vi "JogParams_KCubeInertial.vi"(6 "JogMode in":i32, 9 "JogAcceleration in":i32, 10 "JogRate in":i32, 11 ".NET Refnum in":refnum<k24>) -> (1 "JogAcceleration out":i32, 2 "JogRate out":i32, 3 "JogMode out":i32(ring)=1 items=["Continuous"=1, "Step"=2])   [LabVIEW 2019]
doc: "set and get relative position parameters of inertial motor"
uses:
  D:/Victor Sun/optical trap control/Kinesis/Thorlabs.MotionControl.KCube.InertialMotorCLI.dll
  Kinesis/Thorlabs.MotionControl.KCube.InertialMotorCLI.dll
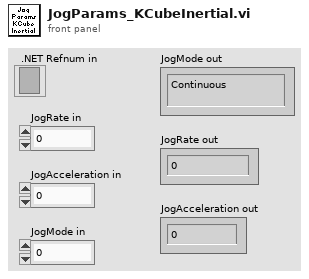
[diagram p1: front panel]
types:
  T1 = cluster{"JogMode":i32, "JogRate":i32, "JogAcceleration":i32}
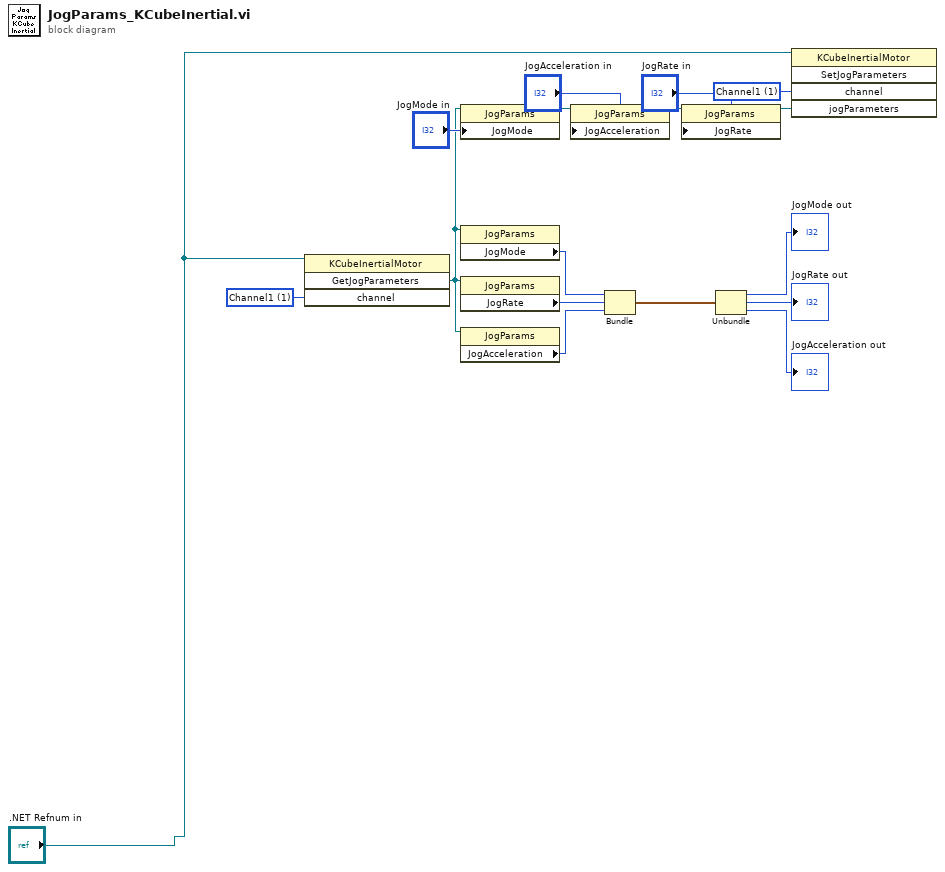
[diagram p0: block diagram]
diagram:
  w5 = 1 items=["Channel1"=1, "Channel2"=2, "Channel3"=3, "Channel4"=4] ("channel")
  w1 = 1 items=["Channel1"=1, "Channel2"=2, "Channel3"=3, "Channel4"=4] ("channel")
  n1 = invoke class="KCubeInertialMotor" method="GetJogParameters"(reference=".NET Refnum in", "channel"=w1) -> ("GetJogParameters"=w6:refnum<k24>)  [unwired: 2 in, 3 out]
  n2 = property class="JogParams"(reference=w6, "JogMode"="JogMode in") -> (reference out=w4:refnum<k24>)  [unwired: 1 in, 1 out]
  n3 = property class="JogParams"(reference=w6) -> ("JogMode"=w8:i32)  [unwired: 1 in, 2 out]
  n4 = property class="JogParams"(reference=w6) -> ("JogRate"=w9:i32)  [unwired: 1 in, 2 out]
  n5 = property class="JogParams"(reference=w6) -> ("JogAcceleration"=w10:i32)  [unwired: 1 in, 2 out]
  n6 = property class="JogParams"(reference=w4, "JogAcceleration"="JogAcceleration in") -> (reference out=w3:refnum<k24>)  [unwired: 1 in, 1 out]
  n7 = Bundle("JogMode"=w8, "JogRate"=w9, "JogAcceleration"=w10) -> (w11:T1)  [unwired: 1 in]
  n8 = property class="JogParams"(reference=w3, "JogRate"="JogRate in") -> (reference out=w2:refnum<k24>)  [unwired: 1 in, 1 out]
  n9 = Unbundle(w11) -> ("JogMode"=→"JogMode out":i32, "JogRate"=→"JogRate out":i32, "JogAcceleration"=→"JogAcceleration out":i32)
  n10 = invoke class="KCubeInertialMotor" method="SetJogParameters"(reference=".NET Refnum in", "channel"=w5, "jogParameters"=w2) -> ()  [unwired: 2 in, 5 out]
